vi "3.1-Parse Act Command.vi"(1 "data out":string) -> (0 "GUI":T1)   [LabVIEW 2010]
uses:
  4-High Neurons/4.1-Act Control Typedef.ctl
  6-OCU Neurons/6.1-UDP Saitek.ctl
  4-High Neurons/4.0-Timing Badass.ctl
  4-High Neurons/6.1-Forbrain Act Neurons.ctl
  4-High Neurons/4.1.2-Act Neuron TD.ctl
  3.0-Global.vi
panel:
  out "data":T2 {"Saitek Controler"."Right" scale=0.0..1.0; "Saitek Controler"."Left" scale=0.0..1.0; "Saitek Controler"."Yaw" scale=-1.0..1.0; "Saitek Controler"."Roll" scale=-1.0..1.0; "Saitek Controler"."Pitch" scale=-1.0..1.0}
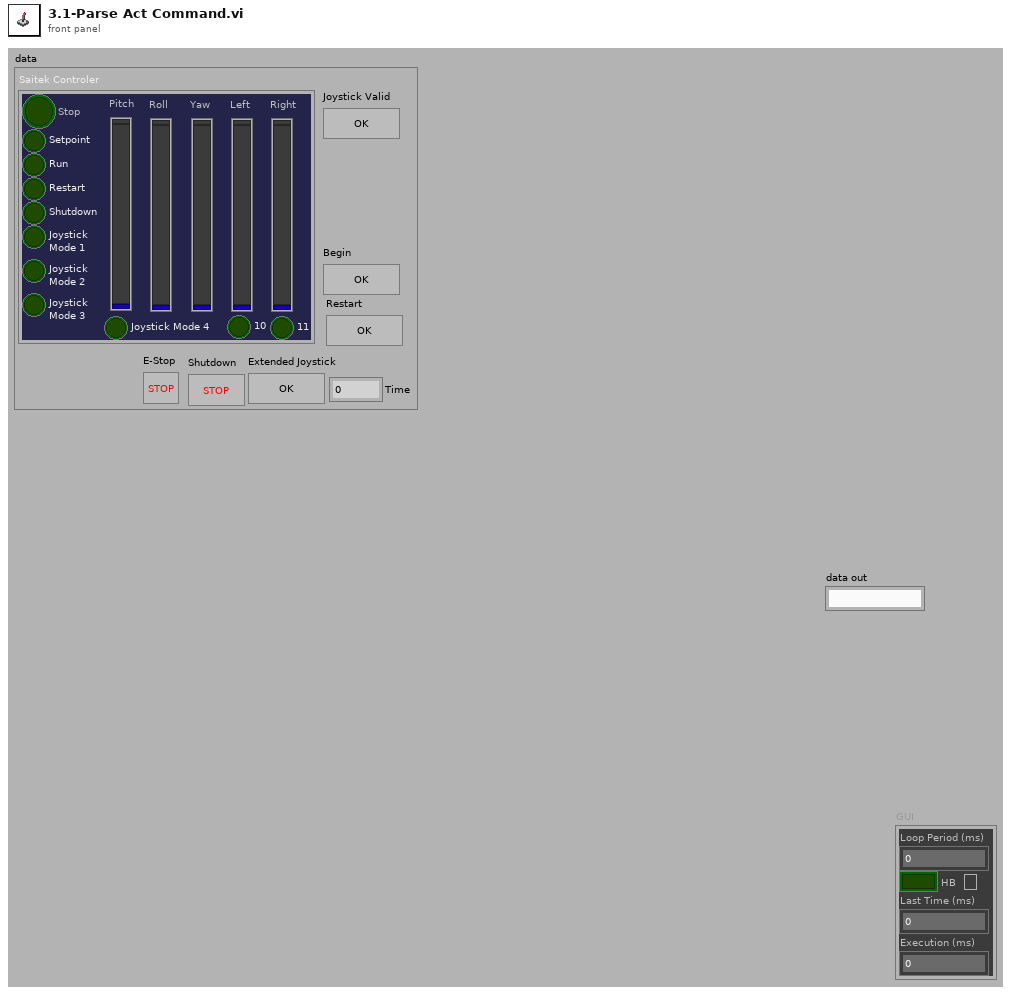
[diagram p1: front panel]
types:
  T1 = typedef "4.0-Timing Badass.ctl" = cluster{"Loop Period (ms)":u32, "HB":bool, "Last Time (ms)":u32, "Execution (ms)":u32}
  T2 = typedef "4.1-Act Control Typedef.ctl" = cluster{"E-Stop":bool, "Restart":bool, "Extended Joystick":bool, "Begin":bool, "Time":i32, "Shutdown":bool, "Saitek Controler":T3, "Joystick Valid":bool}
  T3 = typedef "6.1-UDP Saitek.ctl" = cluster{"Stop":bool, "Setpoint":bool, "Run":bool, "Restart":bool, "Shutdown":bool, "Joystick\nMode 1":bool, "Joystick\nMode 2":bool, "Joystick \nMode 3":bool, "Joystick Mode 4":bool, "10":bool, "11":bool, "Pitch":sgl, "Roll":sgl, "Yaw":sgl, "Left":sgl, "Right":sgl}
  T4 = enum16{"Set Joystick", "Read Joystick", "Set Forebrain", "Read Forebrain", "Set Limbic", "Read Limbic", "Set Cerebellum", "Read Cerebellum", "Set Arbitrated", "Read Arbitrated", "Set LIDAR", "Read LIDAR"}
  T5 = typedef "6.1-Forbrain Act Neurons.ctl" = cluster{"Forebrain Act Neurons":T6, "4.1 Act Control":T2}
  T6 = typedef "4.1.2-Act Neuron TD.ctl" = cluster{"Speed By Path":sgl[]}
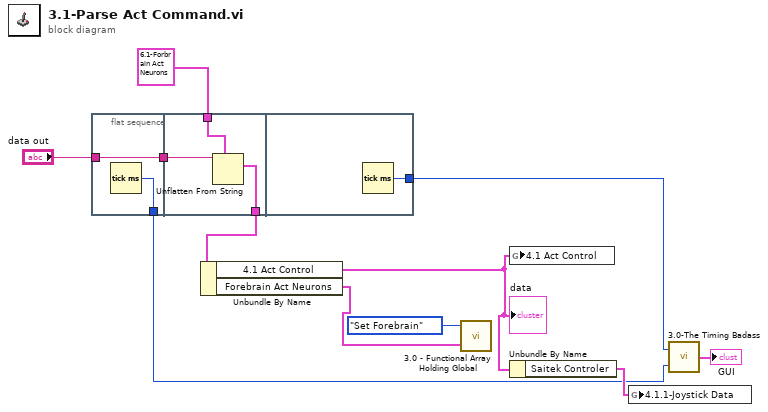
[diagram p0: block diagram]
diagram:
  n1 = flat-sequence {
    tunnel: "data out" -> [w12]
    tunnel: [w13] -> w6
    tunnel: [w12] -> w5
    tunnel: T5 {"Forebrain Act Neurons"={"Speed By Path"=[]}, "4.1 Act Control"={"E-Stop"=FALSE, "Restart"=FALSE, "Extended Joystick"=FALSE, "Begin"=FALSE, "Time"=0, "Shutdown"=FALSE, "Saitek Controler"={"Stop"=FALSE, "Setpoint"=FALSE, "Run"=FALSE, "Restart"=FALSE, "Shutdown"=FALSE, "Joystick\nMode 1"=FALSE, "Joystick\nMode 2"=FALSE, "Joystick \nMode 3"=FALSE, "Joystick Mode 4"=FALSE, "10"=FALSE, "11"=FALSE, "Pitch"=0.0, "Roll"=0.0, "Yaw"=0.0, "Left"=0.0, "Right"=0.0}, "Joystick Valid"=FALSE}} ("6.1-Act Neuron") -> [w15]
    tunnel: w5 -> [w16]
    tunnel: [w14] -> w4
    tunnel: [w17] -> w7
    frame #0 {
      n2 = Tick Count (ms)() -> (millisecond timer value=w13:u32)
    }
    frame #1 {
      n3 = Unflatten From String(type=w15, binary string=w16) -> (value=w14:T5)  [unwired: 3 in, 2 out]
    }
    frame #2 {
      n4 = Tick Count (ms)() -> (millisecond timer value=w17:u32)
    }
  }
  n5 = Unbundle By Name(w4) -> ("4.1 Act Control"=w3:T2, "Forebrain Act Neurons"=w1:T6)
  "data" <- w3
  n6 = call "3.0 - Functional Array Holding Global.vi"("Input Act Neurons"=w1, "Mode"=T4."Set Forebrain") -> ()  [unwired: 1 out]
  n7 = global write "3.0-Global.vi" "4.1 Act Control"(w3) -> ()
  n8 = Unbundle By Name(w3) -> ("Saitek Controler"=w9:T3)
  n9 = global write "3.0-Global.vi" "4.1.1-Joystick Data"(w9) -> ()
  n10 = call "3.0-The Timing Badass.vi"("Start"=w6, "End"=w7) -> ("Super Heart Beat"=→"GUI":T1)
